vi "Get Slave Data.vi"(8 "error in (no error)":errorcluster, 11 "EtherCAT Slave in":T18={"VS ref"=0, "IOV ref"="ni.var.io://localhost/EtherCAT Master/Device", "Position Address"=0} {"VS ref" format="%.0x"}) -> (0 "error out":errorcluster, 3 "EtherCAT Slave out":T1 {"FPGA"."UDVs"."To FPGA"."VS ref" format="%.0x"; "FPGA"."UDVs"."From FPGA"."VS ref" format="%.0x"; "FPGA"."VS ref" format="%.0x"; "FPGA"."Output Data"."BD Refs"."Data Reference" format="%.0x"; "FPGA"."Input Data"."BD Refs"."Data Reference" format="%.0x"; "RSI Modules"."Module Config Data"."Config Block Data Refs"."Data Reference" format="%.0x"; "RSI Modules"."CDOutput Data"."BD Refs"."Data Reference" format="%.0x"; "RSI Modules"."CDInput Data"."BD Refs"."Data Reference" format="%.0x"; "RSI Modules"."VS ref" format="%.0x"; "VS ref" format="%.0x"})   [LabVIEW 2016, in "Scan Engine Custom Device.lvlib"]
uses:
  Scan Engine Custom Device.lvlib
  <vilib>/NI Veristand/Custom Device API/Custom Device Item Ref.ctl
  Type Defs/EtherCAT Slave Data.ctl
  Type Defs/RSI Module Data.ctl
  Type Defs/Open Module IOVs.ctl
  Modules.lvlibp/RSI Module/RSI Module.lvclass
  Modules.lvlibp/RSI Module/Module Models.ctl
  Modules.lvlibp/RSI Module/Channel Type.ctl
  Type Defs/Input Data.ctl
  <vilib>/NI Veristand/Custom Device API/Block Data Reference.ctl
  <vilib>/NI Veristand/Custom Device API/Data Reference.ctl
  Type Defs/Output Data.ctl
  Type Defs/Module Config Data.ctl
  Type Defs/Mixed IO.ctl
  Type Defs/FPGA Data.ctl
  Type Defs/UDV Data.ctl
  Type Defs/UDV Data Type.ctl
  Type Defs/FXP Config.ctl
  Type Defs/Mod Size Indexes.ctl
  <vilib>/NI Veristand/Custom Device API/Custom Device API.lvlib
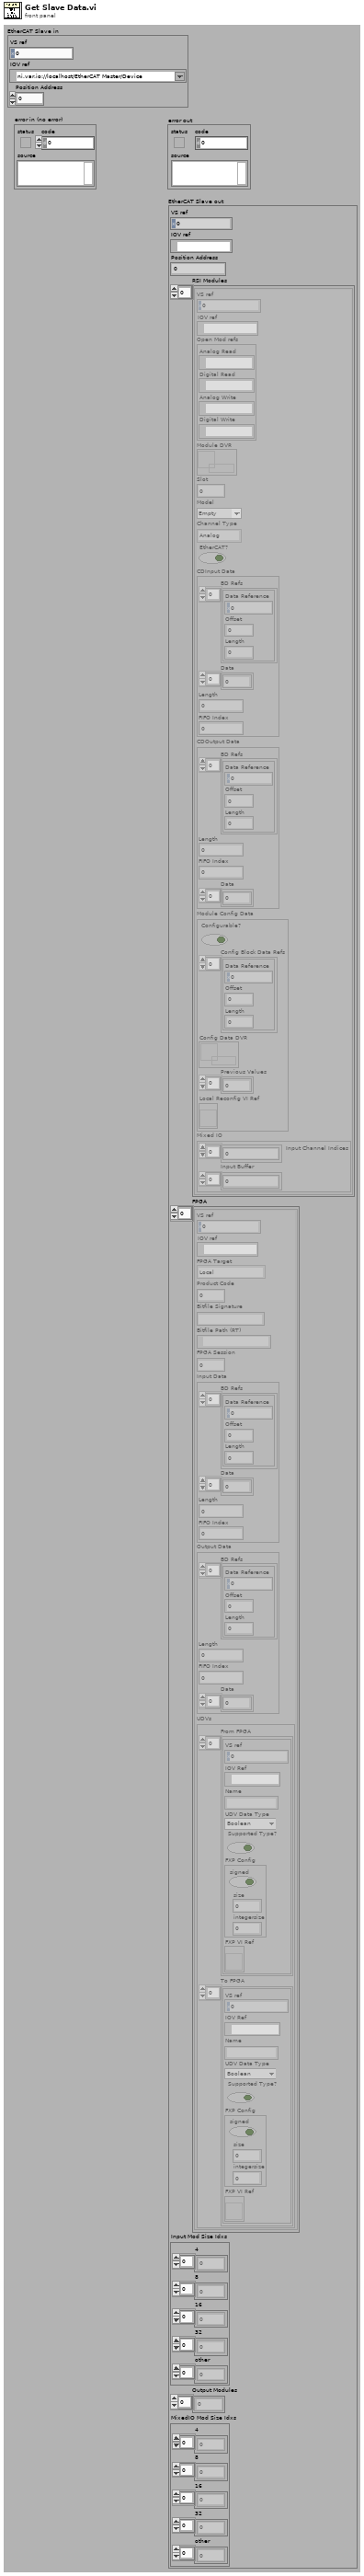
[diagram p1: front panel]
types:
  T1 = typedef "Scan Engine Custom Device.lvlib/EtherCAT Slave Data.ctl" = cluster{"VS ref":T2, "IOV ref":refnum<k21>, "Position Address":u16, "RSI Modules":T3[], "FPGA":T13[], "Input Mod Size Idxs":T17, "Output Modules":i32[], "MixedIO Mod Size Idxs":T17}
  T2 = typedef "Custom Device API.lvlib/Custom Device Item Ref.ctl" = u64
  T3 = typedef "Scan Engine Custom Device.lvlib/RSI Module Data.ctl" = cluster{"VS ref":T2, "IOV ref":refnum<k21>, "Open Mod refs":T4, "Module DVR":refnum<data-value>, "Slot":u32, "Model":T5, "Channel Type":T6, "EtherCAT?":bool, "CDInput Data":T7, "CDOutput Data":T10, "Module Config Data":T11, "Mixed IO":T12}
  T4 = typedef "Scan Engine Custom Device.lvlib/Open Module IOVs.ctl" = cluster{"Analog Read":refnum<k21>, "Digital Read":refnum<k21>, "Analog Write":refnum<k21>, "Digital Write":refnum<k21>}
  T5 = typedef "Modules.lvlibp/RSI Module.lvclass/Module Models.ctl" = enum16{"Empty", "NI 9201", "NI 9203", "NI 9205", "NI 9206", "NI 9207", "NI 9208", "NI 9211", "NI 9212", "NI 9213", "NI 9214", "NI 9215", "NI 9217", "NI 9219", "NI 9220", "NI 9221", "NI 9222", "NI 9223", "NI 9225", "NI 9227", "NI 9229", "NI 9233", "NI 9234", "NI 9235", "NI 9236", "NI 9237", "NI 9239", "NI 9242", "NI 9244", "NI 9263", "NI 9264", "NI 9265", "NI 9269", "NI 9375", "NI 9401", "NI 9402", "NI 9403", "NI 9411", "NI 9421", "NI 9422", "NI 9423", "NI 9425", "NI 9426", "NI 9435", "NI 9437", "NI 9472", "NI 9474", "NI 9475", "NI 9476", "NI 9477", "NI 9478", "NI 9481", "NI 9482", "NI 9485"}
  T6 = typedef "Modules.lvlibp/RSI Module.lvclass/Channel Type.ctl" = enum16{"Analog", "Digital"}
  T7 = typedef "Scan Engine Custom Device.lvlib/Input Data.ctl" = cluster{"BD Refs":T8[], "Data":dbl[], "Length":i32, "FIFO Index":i32}
  T8 = typedef "Custom Device API.lvlib/Block Data Reference.ctl" = cluster{"Data Reference":T9, "Offset":u64, "Length":u64}
  T9 = typedef "Custom Device API.lvlib/Data Reference.ctl" = i32
  T10 = typedef "Scan Engine Custom Device.lvlib/Output Data.ctl" = cluster{"BD Refs":T8[], "Length":i32, "FIFO Index":i32, "Data":dbl[]}
  T11 = typedef "Scan Engine Custom Device.lvlib/Module Config Data.ctl" = cluster{"Configurable?":bool, "Config Block Data Refs":T8[], "Config Data DVR":refnum<data-value>, "Previous Values":dbl[], "Local Reconfig VI Ref":refnum<vi>}
  T12 = typedef "Scan Engine Custom Device.lvlib/Mixed IO.ctl" = cluster{"Input Channel Indices":i32[], "Input Buffer":dbl[]}
  T13 = typedef "Scan Engine Custom Device.lvlib/FPGA Data.ctl" = cluster{"VS ref":T2, "IOV ref":refnum<k21>, "FPGA Target":enum16{"Local", "EtherCAT"}, "Product Code":u32, "Bitfile Signature":string, "Bitfile Path (RT)":path, "FPGA Session":u32, "Input Data":T7, "Output Data":T10, "UDVs":cluster{"From FPGA":T14[], "To FPGA":T14[]}}
  T14 = typedef "Scan Engine Custom Device.lvlib/UDV Data.ctl" = cluster{"VS ref":T2, "IOV Ref":refnum<k21>, "Name":string, "UDV Data Type":T15, "Supported Type?":bool, "FXP Config":T16, "FXP VI Ref":refnum<vi>}
  T15 = typedef "Scan Engine Custom Device.lvlib/UDV Data Type.ctl" = enum16{"Boolean", "Fixed Point", "Int8", "Int16", "Int32", "Int64", "U32 Bit Field", "UInt8", "UInt16", "UInt32", "UInt64", "Other"}
  T16 = typedef "Scan Engine Custom Device.lvlib/FXP Config.ctl" = cluster{"signed":bool, "size":u32, "integersize":i32}
  T17 = typedef "Scan Engine Custom Device.lvlib/Mod Size Indexes.ctl" = cluster{"4":i32[], "8":i32[], "16":i32[], "32":i32[], "other":i32[]}
  T18 = cluster{"VS ref":T2, "IOV ref":refnum<k21>, "Position Address":u16}
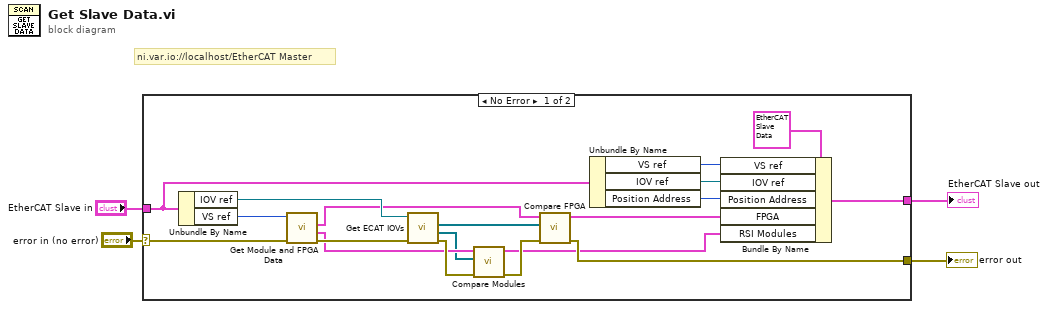
[diagram p0: block diagram]
diagram:
  # "ni.var.io://localhost/EtherCAT Master"
  n1 = case shown="No Error" "error in (no error)" {
    selector: "error in (no error)" -> [w20 w24]
    tunnel: [w15 w24] -> w4
    tunnel: "EtherCAT Slave in" -> [w11 _]
    tunnel: [w5 _] -> w1
    frame No Error {
      n2 = Unbundle By Name(w11) -> ("IOV ref"=w23:refnum<k21>, "VS ref"=w21:T2)
      n3 = call "Get Module and FPGA Data.vi"("error in (no error)"=w20, "Parent Ref in"=w21) -> ("error out"=w19:errorcluster, "RSI Modules"=w18:T3[], "FPGA"=w17:T13[])  [unwired: 5 in, 2 out]
      n4 = call "Get ECAT IOVs.vi"("error in (no error)"=w19, "ECAT Slave in"=w23) -> ("error IO"=w22:errorcluster, "All Mods"=w14:refnum<k21>[], "UDV Container"=w13:refnum<k21>[])  [unwired: 5 in, 2 out]
      n5 = call "Compare Modules.vi"("error in (no error)"=w22, "All Mods"=w14, "RSI Modules in"=w18) -> ("error out"=w16:errorcluster, "RSI Modules out"=w7:T3[])  [unwired: 7 in]
      n6 = call "Compare FPGA.vi"("error in (no error)"=w16, "UDV Container"=w13, "FPGA in"=w17) -> ("error out"=w15:errorcluster, "FPGA out"=w6:T13[])  [unwired: 7 in]
      n7 = Unbundle By Name(w11) -> ("VS ref"=w10:T2, "IOV ref"=w9:refnum<k21>, "Position Address"=w8:u16)
      n8 = Bundle By Name(cluster=T1 {"VS ref"=0, "IOV ref"="", "Position Address"=0, "RSI Modules"=[], "FPGA"=[], "Input Mod Size Idxs"={"4"=[], "8"=[], "16"=[], "32"=[], "other"=[]}, "Output Modules"=[], "MixedIO Mod Size Idxs"={"4"=[], "8"=[], "16"=[], "32"=[], "other"=[]}} ("EtherCAT Slave"), "VS ref"=w10, "IOV ref"=w9, "Position Address"=w8, "FPGA"=w6, "RSI Modules"=w7) -> (w5:T1)
    }
    frame Error {
    }
  }
  "error out" <- w4
  "EtherCAT Slave out" <- w1
